vi "WfmDataAccessor Initialisation.vi"(8 "error in (no error)":errorcluster) -> (0 "error out":errorcluster, 3 "WfmDataAccessor out":refnum<class "WfmDataAccessor.lvclass">)   [LabVIEW 2018, in "WfmDataAccessor.lvclass"]
uses:
  WfmDataAccessor.lvclass
  WfmDataAccessor.lvclass/WfmDataAccessor.ctl
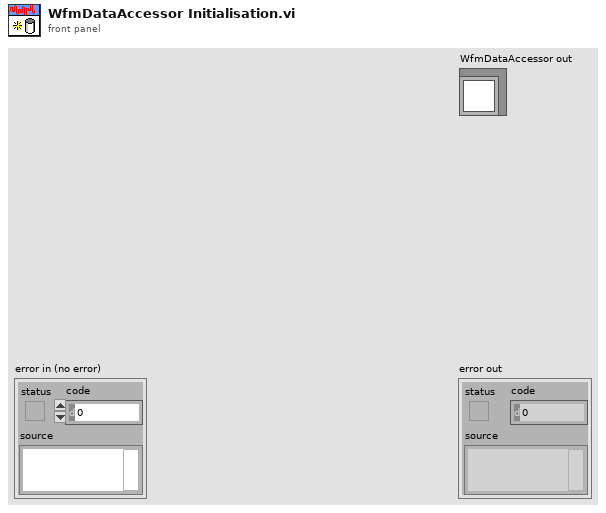
[diagram p1: front panel]
types:
  T1 = enum16{"open", "replace", "create", "open or create", "replace or create", "replace or create with confirmation"}
  T2 = typedef "Semaphore RefNum" = refnum<k1>
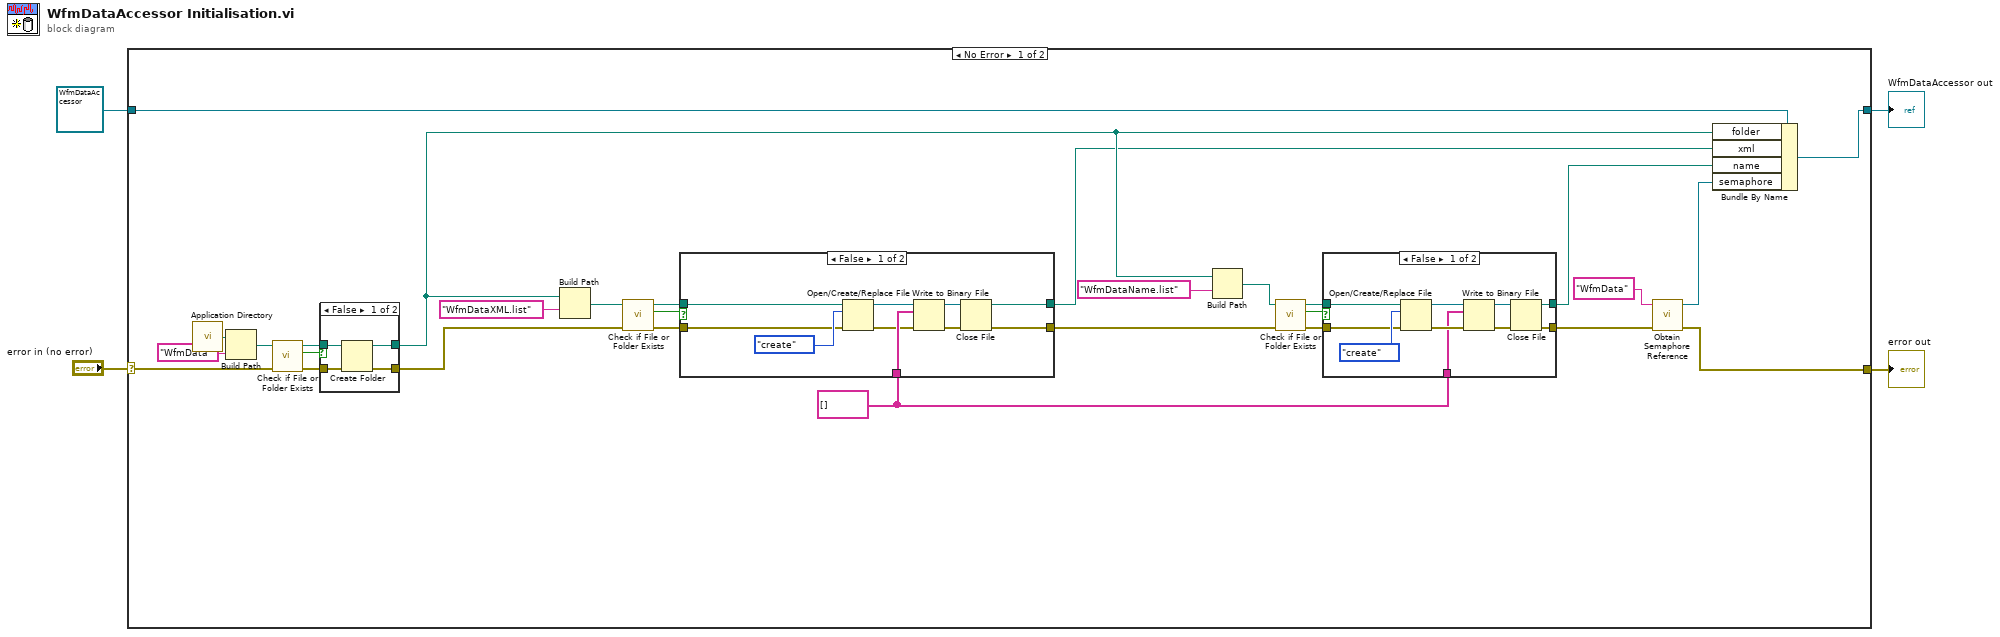
[diagram p0: block diagram]
diagram:
  n1 = case shown="No Error" "error in (no error)" {
    selector: "error in (no error)" -> [w26 w65]
    tunnel: [w5 w65] -> w3
    tunnel: [w24 w64] -> w1
    tunnel: refnum<class "WfmDataAccessor.lvclass"> refnum ("WfmDataAccessor in") -> [w33 w64]
    frame No Error {
      w9 = string[] []
      n2 = call <vilib>:"Application Directory.vi"() -> ("Application Directory"=w27:path)
      n3 = Build Path(base path=w27, name or relative path="WfmData") -> (appended path=w29:path)
      n4 = call <vilib>:"Check if File or Folder Exists.vi"("error in (no error)"=w26, "path"=w29) -> ("error out"=w32:errorcluster, "file or folder exists?"=w30:bool, "dup path"=w31:path)  [unwired: 7 in]
      n5 = case shown="False" w30 {
        tunnel: w31 -> [w61 w63]
        tunnel: w32 -> [w60 w62]
        tunnel: [w59 w63] -> w22
        tunnel: [w58 w62] -> w18
        frame False {
          n6 = Create Folder(path (use dialog)=w61, error in=w60) -> (created path=w59:path, error out=w58:errorcluster)  [unwired: 1 in, 1 out]
        }
        frame True {
        }
      }
      n7 = Build Path(base path=w22, name or relative path="WfmDataXML.list") -> (appended path=w20:path)
      n8 = call <vilib>:"Check if File or Folder Exists.vi"("error in (no error)"=w18, "path"=w20) -> ("error out"=w17:errorcluster, "file or folder exists?"=w16:bool, "dup path"=w19:path)  [unwired: 7 in]
      n9 = case shown="False" w16 {
        tunnel: [w54 w57] -> w21
        tunnel: [w53 w56] -> w14
        tunnel: w19 -> [w50 w57]
        tunnel: w9 -> [w49 _]
        tunnel: w17 -> [w48 w56]
        frame False {
          n10 = Open/Create/Replace File(file path (use dialog)=w50, error in=w48, operation (0:open)=T1."create") -> (refnum out=w47:refnum<file>, error out=w46:errorcluster)  [unwired: 3 in, 1 out]
          n11 = Write to Binary File(file (use dialog)=w47, data=w49, error in=w46) -> (refnum out=w52:refnum<file>, error out=w51:errorcluster)  [unwired: 3 in, 1 out]
          n12 = Close File(refnum=w52, error in=w51) -> (path=w54:path, error out=w53:errorcluster)
        }
        frame True {
        }
      }
      n13 = Build Path(base path=w22, name or relative path="WfmDataName.list") -> (appended path=w15:path)
      n14 = call <vilib>:"Check if File or Folder Exists.vi"("error in (no error)"=w14, "path"=w15) -> ("error out"=w11:errorcluster, "file or folder exists?"=w12:bool, "dup path"=w13:path)  [unwired: 7 in]
      n15 = case shown="False" w12 {
        tunnel: [w41 w45] -> w10
        tunnel: [w40 w44] -> w6
        tunnel: w13 -> [w36 w45]
        tunnel: w9 -> [w35 _]
        tunnel: w11 -> [w34 w44]
        frame False {
          n16 = Open/Create/Replace File(file path (use dialog)=w36, error in=w34, operation (0:open)=T1."create") -> (refnum out=w42:refnum<file>, error out=w38:errorcluster)  [unwired: 3 in, 1 out]
          n17 = Write to Binary File(file (use dialog)=w42, data=w35, error in=w38) -> (refnum out=w39:refnum<file>, error out=w37:errorcluster)  [unwired: 3 in, 1 out]
          n18 = Close File(refnum=w39, error in=w37) -> (path=w41:path, error out=w40:errorcluster)
        }
        frame True {
        }
      }
      n19 = call <vilib>:"Obtain Semaphore Reference.vi"("error in (no error)"=w6, "name (unnamed)"="WfmData") -> ("error out"=w5:errorcluster, "semaphore"=w7:T2)  [unwired: 3 in, 1 out]
      n20 = Bundle By Name(cluster=w33, "folder"=w22, "xml"=w21, "name"=w10, "semaphore"=w7) -> (w24:refnum<class "WfmDataAccessor.lvclass">)
    }
    frame Error {
    }
  }
  "error out" <- w3
  "WfmDataAccessor out" <- w1
